vi "main_feeding.vi"(0 "Env. Ready?":refnum<vi>, 3 "Running?":refnum<vi>, 4 "Selector":refnum<vi>, 5 "Load":refnum<vi>, 6 "Save":refnum<vi>, 7 "Valid?":refnum<vi>, 8 "New Element":refnum<vi>, 9 "Feeding":refnum<vi>, 10 "Delete":refnum<vi>, 11 "Add":refnum<vi>) -> (2 "timetable":string)   [LabVIEW 2019]
uses:
  lib/libFileFunctions/libFileFunctions.lvlib
  lib/libSimulationControl/libSimulationControl.lvlib
panel:
  out "hydro_path":path
  out "Timetable arr":string[][](array[string])
  # "*******************************************************************\nBiogas Plant Control\n\nAuthor: Paul Zügel\nGCSC-Frankfurt am Main 2020\n\n*******************************************************************"
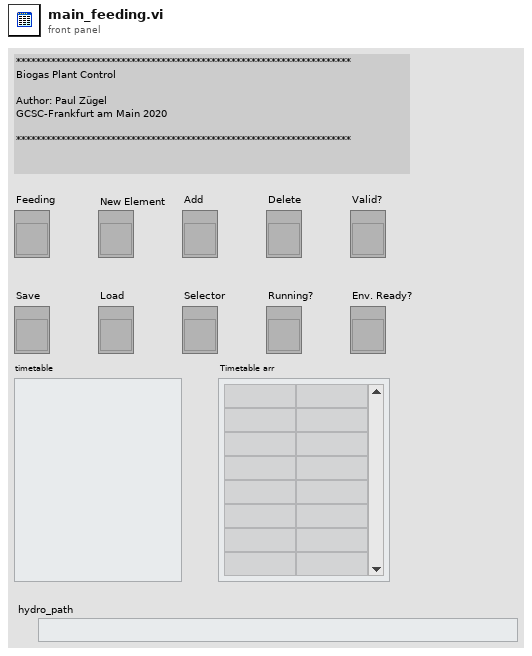
[diagram p1: front panel]
types:
  T1 = enum8{"Enabled", "Disabled", "Disabled and Grayed Out"}
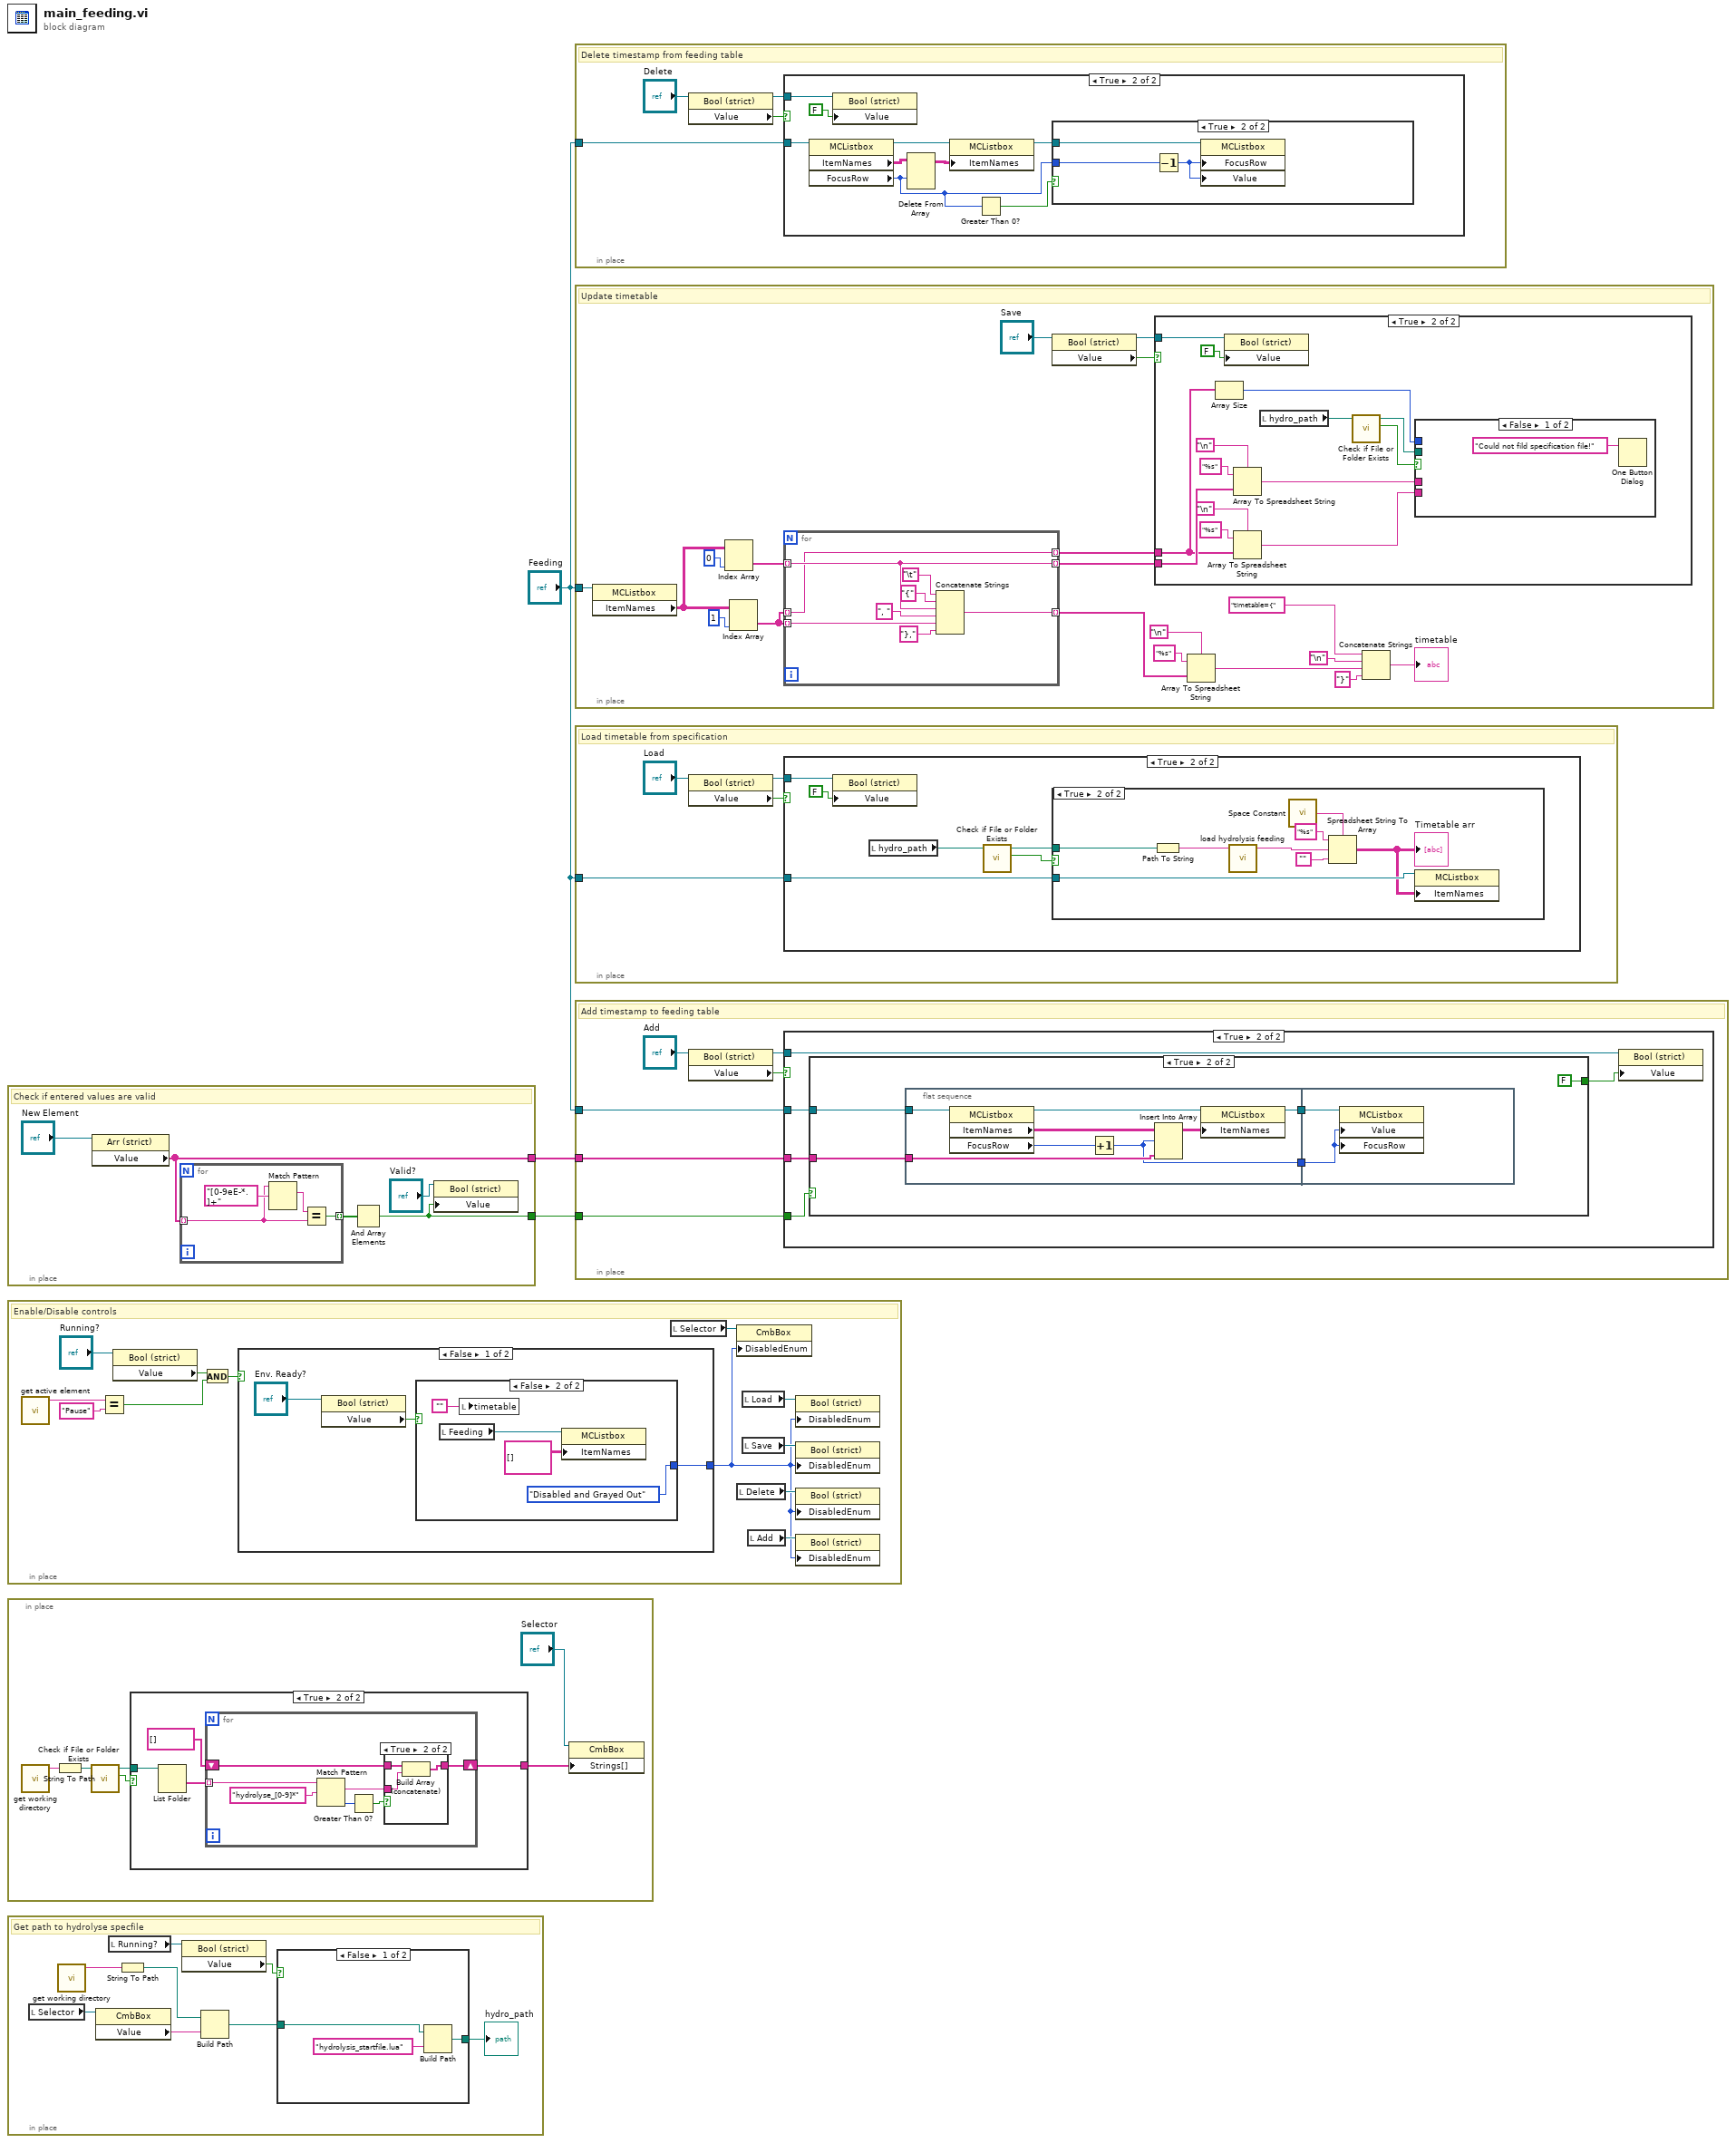
[diagram p0: block diagram]
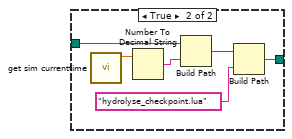
[diagram p2: hidden frame]
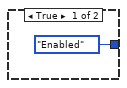
[diagram p3: hidden frame]
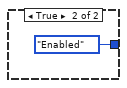
[diagram p4: hidden frame]
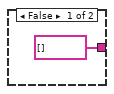
[diagram p5: hidden frame]
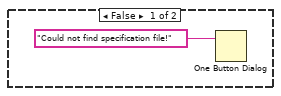
[diagram p8: hidden frame]
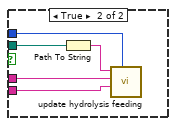
[diagram p10: hidden frame]
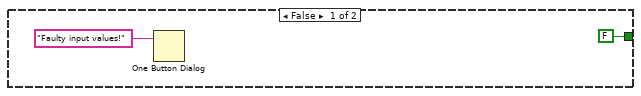
[diagram p14: hidden frame]
diagram:
  n1 = in-place {
    in-place-border: [w6] -> w3
    in-place-border: [w4] -> w2
    # "Check if entered values are valid"
    n2 = property class="Arr (strict)"(reference="New Element") -> ("Value"=w6:string[])  [unwired: 1 in, 2 out]
    n3 = for {
      tunnel: w6 -> [w10] mode=indexing
      tunnel: [w9] -> w7 mode=indexing
      n4 = Match Pattern(string=w10, regular expression="[0-9eE-*.]+") -> (match substring=w12:string)  [unwired: 1 in, 3 out]
      n5 = Equal?(x=w12, y=w10) -> (x = y?=w9:bool)
    }
    n6 = And Array Elements(Boolean array=w7) -> (logical AND=w4:bool)
    n7 = property on="Property Node" class="Bool (strict)"(reference="Valid?", "Value"=w4) -> ()  [unwired: 1 in, 2 out]
  }
  n8 = in-place {
    # "Enable/Disable controls"
    n9 = call "get active element.vi"() -> ("active_element"=w23:string)  [unwired: 10 in, 1 out]
    n10 = Equal?(x=w23, y="Pause") -> (x = y?=w20:bool)
    n11 = property class="Bool (strict)"(reference="Running?") -> ("Value"=w21:bool)  [unwired: 1 in, 2 out]
    n12 = And(x=w21, y=w20) -> (x .and. y?=w19:bool)
    n13 = case shown="False" w19 {
      tunnel: [w27 T1."Enabled" ("Disabled")] -> w13
      frame False {
        n14 = property class="Bool (strict)"(reference="Env. Ready?") -> ("Value"=w25:bool)  [unwired: 1 in, 2 out]
        n15 = case shown="False" w25 {
          tunnel: [T1."Enabled" ("Disabled") T1."Disabled and Grayed Out" ("Disabled")] -> w27
          frame True {
          }
          frame False {
            n16 = local read "Feeding"() -> (w31:refnum<vi>)
            n17 = local write "timetable"("") -> ()
            n18 = property class="MCListbox"(reference=w31, "ItemNames"=string[][] [] ("Item Names")) -> ()  [unwired: 1 in, 2 out]
          }
        }
      }
      frame True {
      }
    }
    n19 = local read "Selector"() -> (w15:refnum<vi>)
    n20 = property class="CmbBox"(reference=w15, "DisabledEnum"=w13) -> ()  [unwired: 1 in, 2 out]
    n21 = local read "Delete"() -> (w16:refnum<vi>)
    n22 = local read "Load"() -> (w17:refnum<vi>)
    n23 = local read "Save"() -> (w14:refnum<vi>)
    n24 = local read "Add"() -> (w18:refnum<vi>)
    n25 = property class="Bool (strict)"(reference=w17, "DisabledEnum"=w13) -> ()  [unwired: 1 in, 2 out]
    n26 = property class="Bool (strict)"(reference=w14, "DisabledEnum"=w13) -> ()  [unwired: 1 in, 2 out]
    n27 = property class="Bool (strict)"(reference=w16, "DisabledEnum"=w13) -> ()  [unwired: 1 in, 2 out]
    n28 = property class="Bool (strict)"(reference=w18, "DisabledEnum"=w13) -> ()  [unwired: 1 in, 2 out]
  }
  n29 = in-place {
    n30 = call "get working directory.vi"() -> ("function return"=w39:string)  [unwired: 10 in, 1 out]
    n31 = String To Path(string=w39) -> (path=w36:path)
    n32 = call <vilib>:"Check if File or Folder Exists.vi"("path"=w36) -> ("file or folder exists?"=w34:bool, "dup path"=w35:path)  [unwired: 8 in, 1 out]
    n33 = case shown="True" w34 {
      tunnel: w35 -> [_ w42]
      tunnel: [string[] [] w41] -> w37
      frame False {
      }
      frame True {
        n34 = List Folder(path=w42) -> (folder names=w44:string[])  [unwired: 3 in, 3 out]
        n35 = for {
          tunnel: w44 -> [w45] mode=indexing
          shift-right: [w46] -> w41
          shift-left: string[] [] -> [w48]
          n36 = Match Pattern(string=w45, regular expression="hydrolyse_[0-9]*") -> (match substring=w47:string, offset past match=w49:i32)  [unwired: 1 in, 2 out]
          n37 = Greater Than 0?(x=w49) -> (x > 0?=w50:bool)
          n38 = case shown="True" w50 {
            tunnel: [w52 w55] -> w46
            tunnel: w48 -> [w52 w54]
            tunnel: w47 -> [_ w53]
            frame False {
            }
            frame True {
              n39 = Build Array (concatenate)(w54, w53) -> (w55:string[])
            }
          }
        }
      }
    }
    n40 = property class="CmbBox"(reference="Selector", "Strings[]"=w37) -> ()  [unwired: 1 in, 2 out]
  }
  n41 = in-place {
    # "Get path to hydrolyse specfile"
    n42 = local read "Selector"() -> (w63:refnum<vi>)
    n43 = call "get working directory.vi"() -> ("function return"=w62:string)  [unwired: 10 in, 1 out]
    n44 = property class="CmbBox"(reference=w63) -> ("Value"=w60:string)  [unwired: 1 in, 2 out]
    n45 = local read "Running?"() -> (w57:refnum<vi>)
    n46 = String To Path(string=w62) -> (path=w61:path)
    n47 = property class="Bool (strict)"(reference=w57) -> ("Value"=w56:bool)  [unwired: 1 in, 2 out]
    n48 = Build Path(base path=w61, name or relative path=w60) -> (appended path=w59:path)
    n49 = case shown="False" w56 {
      tunnel: w59 -> [w66 w72]
      tunnel: [w65 w67] -> w58
      frame False {
        n50 = Build Path(base path=w66, name or relative path="hydrolysis_startfile.lua") -> (appended path=w65:path)
      }
      frame True {
        n51 = call "get sim currenttime.vi"() -> ("current_time"=w71:dbl)  [unwired: 10 in, 1 out]
        n52 = Number To Decimal String(number=w71) -> (decimal integer string=w70:string)  [unwired: 1 in]
        n53 = Build Path(base path=w72, name or relative path=w70) -> (appended path=w69:path)
        n54 = Build Path(base path=w69, name or relative path="hydrolyse_checkpoint.lua") -> (appended path=w67:path)
      }
    }
    "hydro_path" <- w58
  }
  n55 = in-place {
    in-place-border: "Feeding" -> [w76]
    # "Delete timestamp from feeding table"
    n56 = property on="Property Node" class="Bool (strict)"(reference="Delete") -> (reference out=w75:refnum<vi>, "Value"=w74:bool)  [unwired: 1 in, 1 out]
    n57 = case shown="True" w74 {
      tunnel: w76 -> [_ w85]
      tunnel: w75 -> [_ w83]
      frame False {
      }
      frame True {
        n58 = property on="Property Node" class="MCListbox"(reference=w85) -> (reference out=w80:refnum<vi>, "ItemNames"=w82:string[][], "FocusRow"=w78:i32)  [unwired: 1 in, 1 out]
        n59 = property on="Property Node" class="Bool (strict)"(reference=w83, "Value"=FALSE) -> ()  [unwired: 1 in, 2 out]
        n60 = Delete From Array(array=w82, index (row)=w78) -> (array with subset deleted=w81:string[][])  [unwired: 2 in, 1 out]
        n61 = property on="Property Node" class="MCListbox"(reference=w80, "ItemNames"=w81) -> (reference out=w84:refnum<vi>)  [unwired: 1 in, 1 out]
        n62 = Greater Than 0?(x=w78) -> (x > 0?=w77:bool)
        n63 = case shown="True" w77 {
          tunnel: w78 -> [_ w88]
          tunnel: w84 -> [_ w87]
          frame False {
          }
          frame True {
            n64 = Decrement(x=w88) -> (x-1=w86:i32)
            n65 = property on="Property Node" class="MCListbox"(reference=w87, "FocusRow"=w86, "Value"=w86) -> ()  [unwired: 1 in, 2 out]
          }
        }
      }
    }
  }
  n66 = in-place {
    in-place-border: "Feeding" -> [w100]
    # "Update timetable"
    n67 = property on="Property Node" class="MCListbox"(reference=w100) -> ("ItemNames"=w101:string[][])  [unwired: 1 in, 2 out]
    n68 = Index Array(array=w101, index (col)=0 ("disabled index (col)")) -> (element=w103:string[])  [unwired: 1 in]
    n69 = Index Array(array=w101, index (col)=1 ("disabled index (col)")) -> (element=w91:string[])  [unwired: 1 in]
    n70 = for {
      tunnel: w103 -> [w129] mode=indexing
      tunnel: w91 -> [w130] mode=indexing
      tunnel: [w135] -> w102 mode=indexing
      tunnel: [w128] -> w92 mode=indexing
      tunnel: [w129] -> w90 mode=indexing
      tunnel: w91 -> [w128] mode=indexing
      n71 = Concatenate Strings("\t", "{" ("string"), w129, ", " ("string"), w130, "}," ("string")) -> (w135:string)
    }
    n72 = property class="Bool (strict)"(reference="Save") -> (reference out=w89:refnum<vi>, "Value"=w94:bool)  [unwired: 1 in, 1 out]
    n73 = case shown="True" w94 {
      tunnel: w92 -> [_ w114]
      tunnel: w90 -> [_ w120]
      tunnel: w89 -> [_ w112]
      frame False {
      }
      frame True {
        n74 = Array Size(array=w114) -> (size(s)=w121:i32)
        n75 = property class="Bool (strict)"(reference=w112, "Value"=FALSE) -> ()  [unwired: 1 in, 2 out]
        n76 = Array To Spreadsheet String(delimiter (Tab)="\n", array=w120, 3:"%s" ("format string")) -> (spreadsheet string=w117:string)
        n77 = Array To Spreadsheet String(delimiter (Tab)="\n", array=w114, 3:"%s" ("format string")) -> (spreadsheet string=w113:string)
        n78 = local read "hydro_path"() -> (w110:path)
        n79 = call <vilib>:"Check if File or Folder Exists.vi"("path"=w110) -> ("file or folder exists?"=w109:bool, "dup path"=w108:path)  [unwired: 8 in, 1 out]
        n80 = case shown="False" w109 {
          tunnel: w121 -> [_ w127]
          tunnel: w117 -> [_ w126]
          tunnel: w113 -> [_ w125]
          tunnel: w108 -> [_ w124]
          frame False {
            n81 = One Button Dialog(message="Could not fild specification file!") -> ()  [unwired: 1 in, 1 out]
          }
          frame True {
            n82 = Path To String(path=w124) -> (string=w123:string)
            n83 = call "update hydrolysis feeding.vi"("number_timestamps"=w127, "amount"=w125, "time"=w126, "hydrolysis_specfile"=w123) -> ()  [unwired: 7 in, 1 out]
          }
        }
      }
    }
    n84 = Array To Spreadsheet String(delimiter (Tab)="\n", array=w102, 3:"%s" ("format string")) -> (spreadsheet string=w97:string)
    n85 = Concatenate Strings("timetable={" ("string"), "\n", w97, "}" ("string")) -> (→"timetable":string)
  }
  n86 = in-place {
    in-place-border: "Feeding" -> [w139]
    # "Load timetable from specification"
    n87 = property on="Property Node" class="Bool (strict)"(reference="Load") -> (reference out=w136:refnum<vi>, "Value"=w137:bool)  [unwired: 1 in, 1 out]
    n88 = case shown="True" w137 {
      tunnel: w139 -> [_ w145]
      tunnel: w136 -> [_ w144]
      frame False {
      }
      frame True {
        n89 = property on="Property Node" class="Bool (strict)"(reference=w144, "Value"=FALSE) -> ()  [unwired: 1 in, 2 out]
        n90 = local read "hydro_path"() -> (w142:path)
        n91 = call <vilib>:"Check if File or Folder Exists.vi"("path"=w142) -> ("file or folder exists?"=w141:bool, "dup path"=w140:path)  [unwired: 8 in, 1 out]
        n92 = case shown="True" w141 {
          tunnel: w145 -> [_ w154]
          tunnel: w140 -> [_ w148]
          frame False {
            n93 = One Button Dialog(message="Could not find specification file!") -> ()  [unwired: 1 in, 1 out]
          }
          frame True {
            n94 = Path To String(path=w148) -> (string=w147:string)
            n95 = call "load hydrolysis feeding.vi"("hydrolysis_specfile"=w147) -> ("function return"=w153:string)  [unwired: 9 in, 1 out]
            n96 = call <vilib>:"Space Constant.vi"() -> ("String"=w149:string)
            n97 = Spreadsheet String To Array(delimiter (Tab)=w149, format string="%s", spreadsheet string=w153, array type (2D Dbl)="") -> (array=w150:string[][])
            "Timetable arr" <- w150
            n98 = property class="MCListbox"(reference=w154, "ItemNames"=w150) -> ()  [unwired: 1 in, 2 out]
          }
        }
      }
    }
  }
  n99 = in-place {
    in-place-border: "Feeding" -> [w160]
    in-place-border: w3 -> [w157]
    in-place-border: w2 -> [w156]
    # "Add timestamp to feeding table"
    n100 = property class="Bool (strict)"(reference="Add") -> (reference out=w158:refnum<vi>, "Value"=w159:bool)  [unwired: 1 in, 1 out]
    n101 = case shown="True" w159 {
      tunnel: w160 -> [_ w165]
      tunnel: w158 -> [_ w163]
      tunnel: w157 -> [_ w162]
      tunnel: w156 -> [_ w161]
      frame False {
      }
      frame True {
        n102 = case shown="True" w161 {
          tunnel: w162 -> [_ w172]
          tunnel: w165 -> [_ w170]
          tunnel: [FALSE ("Value") FALSE ("Value")] -> w164
          frame False {
            n103 = One Button Dialog(message="Faulty input values!") -> ()  [unwired: 1 in, 1 out]
          }
          frame True {
            n104 = flat-sequence {
              tunnel: w172 -> [w180]
              tunnel: [w177] -> w171
              tunnel: w170 -> [w175]
              tunnel: [w173] -> w169
              tunnel: w171 -> [w182]
              tunnel: w169 -> [w181]
              frame #0 {
                n105 = property on="Property Node" class="MCListbox"(reference=w175) -> (reference out=w174:refnum<vi>, "ItemNames"=w179:string[][], "FocusRow"=w176:i32)  [unwired: 1 in, 1 out]
                n106 = Increment(x=w176) -> (x+1=w177:i32)
                n107 = Insert Into Array(array=w179, index (row)=w177, new element=w180) -> (w178:string[][])  [unwired: 1 in]
                n108 = property on="Property Node" class="MCListbox"(reference=w174, "ItemNames"=w178) -> (reference out=w173:refnum<vi>)  [unwired: 1 in, 1 out]
              }
              frame #1 {
                n109 = property on="Property Node" class="MCListbox"(reference=w181, "Value"=w182, "FocusRow"=w182) -> ()  [unwired: 1 in, 2 out]
              }
            }
          }
        }
        n110 = property class="Bool (strict)"(reference=w163, "Value"=w164) -> ()  [unwired: 1 in, 2 out]
      }
    }
  }
